vi "ValuesExtract.vi"(1 "Indication voulue":string, 2 "Chaine de caractères":string) -> (0 "Resulta":dbl)   [LabVIEW 2018]
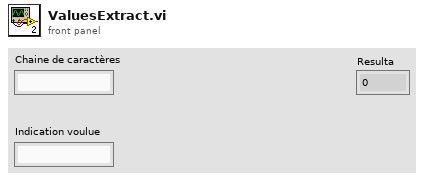
[diagram p1: front panel]
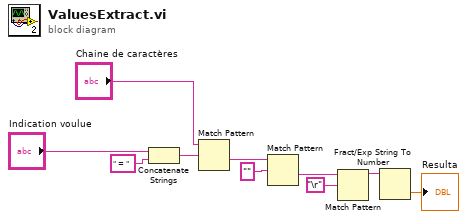
[diagram p0: block diagram]
diagram:
  n1 = Concatenate Strings("Indication voulue", " = " ("string")) -> (w8:string)
  n2 = Match Pattern(string="Chaine de caractères", regular expression=w8) -> (after substring=w5:string)  [unwired: 1 in, 3 out]
  n3 = Match Pattern(string=w5, regular expression="") -> (after substring=w4:string)  [unwired: 1 in, 3 out]
  n4 = Match Pattern(string=w4, regular expression="\r") -> (before substring=w2:string)  [unwired: 1 in, 3 out]
  n5 = Fract/Exp String To Number(string=w2) -> (number=→"Resulta":dbl)  [unwired: 3 in, 1 out]
